vi "Result Response.vi"(8 "error in (no error)":errorcluster, 10 "Acquired Result.lvclass":refnum<class "Acquired Result.lvclass">, 11 "Monitor Controller in":refnum<class "Monitor Controller.lvclass">) -> (0 "error out":errorcluster, 3 "Monitor Controller out":refnum<class "Monitor Controller.lvclass">)   [LabVIEW 2016, in "Monitor Controller.lvclass"]
uses:
  Monitor Controller.lvclass
  C:/github/LabActor/Worker/Worker.lvclass
  C:/Program Files/National Instruments/LabVIEW 2016/vi.lib/ActorFramework/Actor/Actor.lvclass
  NHMFL_Core/Libraries/Instruments/Results/Acquired Result/Acquired Result.lvclass
  Worker/Worker.lvclass/Worker.ctl
  Monitor Controller.lvclass/Monitor Controller.ctl
  <vilib>/ActorFramework/Actor/Actor.lvclass/Actor.ctl
  Process Controller Messages/Update Plots Msg/Update Plots Msg.lvclass/Update Plots Msg.ctl
  <vilib>/ActorFramework/Message Enqueuer/Message Enqueuer.lvclass/Message Enqueuer.ctl
  Worker/Read File Path.vi
  <vilib>/ActorFramework/Message Enqueuer/Enqueue.vi
  Process Controller Messages/Update Plots Msg/Update Plots Msg.lvclass
  C:/Program Files/National Instruments/LabVIEW 2016/vi.lib/ActorFramework/Message/Message.lvclass
  Read Monitor controller configuration.vi
  <vilib>/ActorFramework/Message Priority Queue/Priority Enqueue.vi
  Process Controller/Process Controller.lvclass
  <vilib>/ActorFramework/Actor/Actor.lvclass
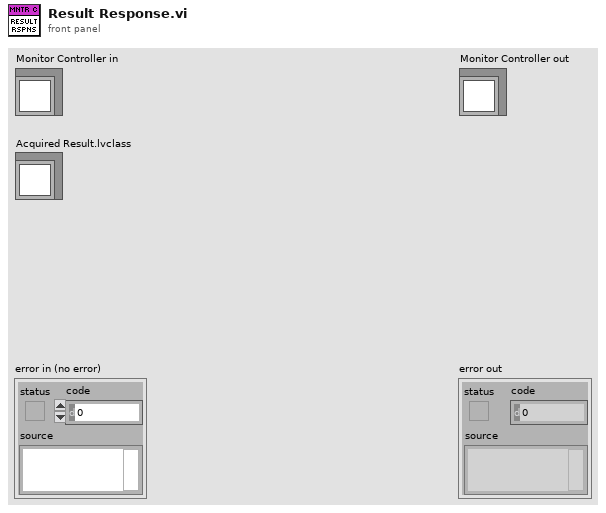
[diagram p1: front panel]
types:
  T1 = typedef "Monitor Controller Configuration.ctl" = cluster{"Update period":dbl, "Repeat times":i32, "Open plot":bool, "File defragment period":dbl, "Timestamp data points":bool, "Re-plot rate limit":dbl}
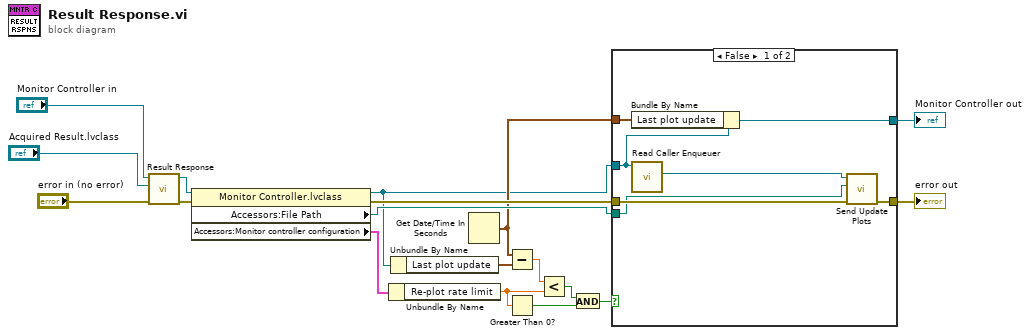
[diagram p0: block diagram]
diagram:
  n1 = call-parent "Result Response.vi"("error in (no error)"="error in (no error)", "Acquired Result"="Acquired Result.lvclass", "Measure Controller in"="Monitor Controller in") -> ("error out"=w12:errorcluster, "Measure Controller out"=w15:refnum<class "Monitor Controller.lvclass">)  [unwired: 7 in]
  n2 = property class="Monitor Controller.lvclass"(reference=w15, error in=w12) -> (reference out=w2:refnum<class "Monitor Controller.lvclass">, error out=w14:errorcluster, "Accessors:File Path"=w11:path, "Accessors:Monitor controller configuration"=w10:T1)
  n3 = Unbundle By Name(w10) -> ("Re-plot rate limit"=w6:dbl)
  n4 = Unbundle By Name(w2) -> ("Last plot update"=w9:timestamp)
  n5 = Get Date/Time In Seconds() -> (seconds since 1Jan1904=w3:timestamp)
  n6 = Subtract(x=w3, y=w9) -> (x-y=w8:dbl)
  n7 = Greater Than 0?(x=w6) -> (x > 0?=w7:bool)
  n8 = Less?(x=w8, y=w6) -> (x < y?=w5:bool)
  n9 = And(x=w5, y=w7) -> (x .and. y?=w4:bool)
  n10 = case shown="False" w4 {
    tunnel: w2 -> [w21 w26]
    tunnel: w14 -> [w24 w27]
    tunnel: [w23 w27] -> w13
    tunnel: w11 -> [w22 _]
    tunnel: w3 -> [w20 _]
    tunnel: [w19 w26] -> w1
    frame False {
      n11 = Bundle By Name(cluster=w21, "Last plot update"=w20) -> (w19:refnum<class "Monitor Controller.lvclass">)
      n12 = call <vilib>:"Read Caller Enqueuer.vi"("Actor"=w21) -> ("Caller Enqueuer"=w25:refnum<class "Message Enqueuer.lvclass">)  [unwired: 10 in]
      n13 = call "Send Update Plots.vi"("error in (no error)"=w24, "File Path"=w22, "Message Enqueuer"=w25) -> ("error out"=w23:errorcluster)  [unwired: 7 in, 1 out]
    }
    frame True {
      # "Wait untill rate limit elapsed"
    }
  }
  "error out" <- w13
  "Monitor Controller out" <- w1
